vi "SetConfigurationString.vi"(8 "Error In":errorcluster, 9 "String":string, 10 "Identification":string, 11 "reference in":refnum<class "IApplicationConfiguration.lvclass">) -> (0 "Error Out":errorcluster, 3 "reference out":refnum<class "IApplicationConfiguration.lvclass">)   [LabVIEW 2021, in "IApplicationConfiguration.lvclass"]
uses:
  IApplicationConfiguration.lvclass
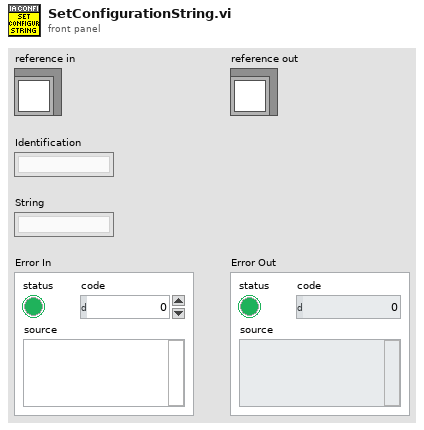
[diagram p1: front panel]
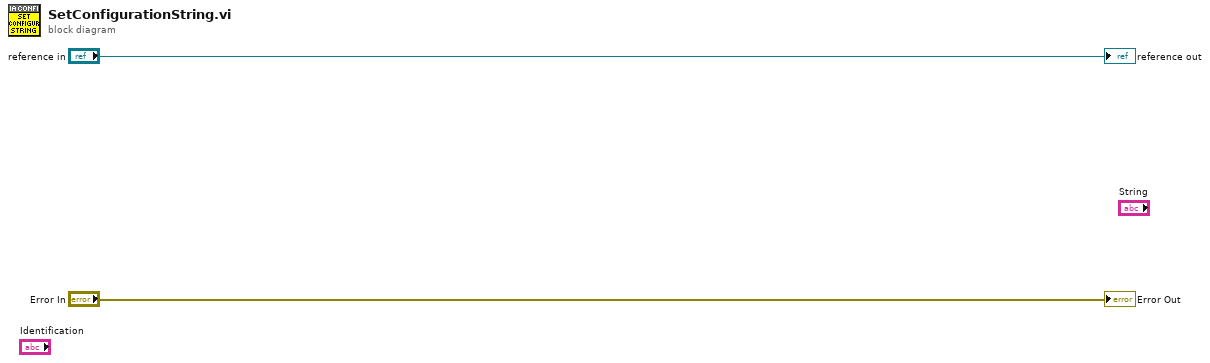
[diagram p0: block diagram]
diagram:
  "Error Out" <- "Error In"
  "reference out" <- "reference in"
